vi "DSF.Memory.Pointer.Channel Properties.Read.0D.vi"(8 "error in (no error)":errorcluster, 10 "channel index":u64, 11 "Channel Properties Pointer in":refnum<class "DSF.Memory.Pointer.Channel Properties.lvclass">) -> (0 "error out":errorcluster, 1 "channel properties":T1 {"size" format="%d bytes"; "offset" format="%d bytes"}, 3 "Channel Properties Pointer out":refnum<class "DSF.Memory.Pointer.Channel Properties.lvclass">)   [LabVIEW 2016, in "DSF.Memory.lvlib" / "DSF.Memory.Pointer.Channel Properties.lvclass"]
uses:
  DSF.Memory.Pointer.Channel Properties.lvclass
  C:/Git/SourceTree/DSF/Source/Classes/Memory.Pointer.Array/DSF.Memory.Pointer.Array.lvclass
  C:/Git/SourceTree/DSF/Source/Submodules/Memory Manager/Source/Classes/Pointer/Memory.Pointer.lvclass
  Typedefs/DSF.Common.Channel Properties.ctl
  Typedefs/DSF.Common.DataType.ctl
  Memory.Pointer.Array/DSF.Memory.Pointer.Array.lvclass/DSF.Memory.Pointer.Array.ctl
  Submodules/Memory Manager/Source/Classes/Pointer/Memory.Pointer.lvclass/Memory.Pointer.ctl
  Submodules/Memory Manager/Source/Classes/Pointer/Methods/Memory.Pointer.Errors.vi
  Submodules/Memory Manager/Source/Classes/Pointer/Methods/Memory.Pointer.Errors.Out of Bounds.vi
  Submodules/Memory Manager/Source/Classes/Pointer/Accessors/Get Size.vi
  Submodules/Memory Manager/Source/Submodules/SEH/Source/VIs/Static Error Handling.Source Buffer.Write.String.vi
  Submodules/Memory Manager/Source/Classes/Pointer/Methods/Memory.Pointer.Errors.Write Pointer Size.vi
  Submodules/Memory Manager/Source/Classes/Pointer/Methods/Memory.Pointer.Errors.Create Error.vi
  Submodules/Memory Manager/Source/Submodules/SEH/Source/VIs/Static Error Handling.Source Buffer.Write.Numeric.Scalar.Base10.vi
  Submodules/Memory Manager/Source/Submodules/SEH/Source/VIs/Static Error Handling.Source Buffer.Write.Numeric.Scalar.Base10 (U64).vi
  Submodules/Memory Manager/Source/Submodules/SEH/Source/VIs/Static Error Handling.Error Cluster Constant.vi
  Submodules/Memory Manager/Source/Submodules/SEH/Source/VIs/Static Error Handling.Error Cluster Constant (256B).vi
  Submodules/Memory Manager/Source/Submodules/SEH/Source/VIs/Static Error Handling.Parameters.Status.Set.vi
  Submodules/Memory Manager/Source/Submodules/SEH/Source/VIs/Static Error Handling.Parameters.Code.Set.vi
  Submodules/Memory Manager/Source/Submodules/SEH/Source/VIs/Static Error Handling.Parameters.VI Source.Set.vi
  Submodules/Memory Manager/Source/Constants/Memory.Constants.vi
  Submodules/Memory Manager/Source/Constants/Memory.Constants.Library Name.vi
  Submodules/Memory Manager/Source/Classes/Pointer/Methods/Memory.Pointer.Errors.Get Info.vi
  Memory.Pointer.Array/DSF.Memory.Pointer.Array.lvclass
  Submodules/Memory Manager/Source/Classes/Pointer/Memory.Pointer.lvclass
  DSF.Common.lvlib
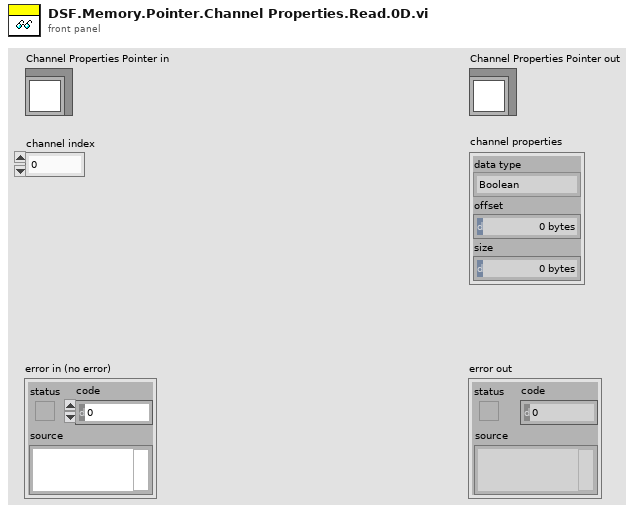
[diagram p1: front panel]
types:
  T1 = typedef "DSF.Common.lvlib/DSF.Common.Channel Properties.ctl" = cluster{"data type":T2, "offset":u64, "size":u64}
  T2 = typedef "DSF.Common.lvlib/DSF.Common.DataType.ctl" = enum8{"Boolean", "Single", "Double", "Int8", "Int16", "Int32", "Int64", "UInt8", "UInt16", "UInt32", "UInt64"}
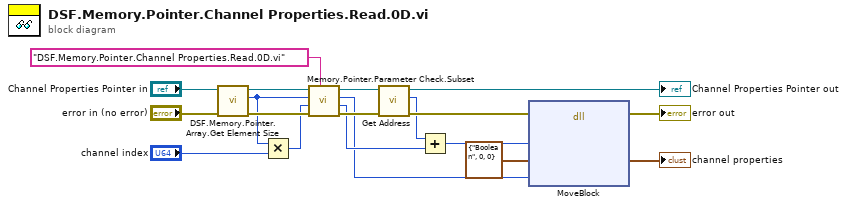
[diagram p0: block diagram]
diagram:
  n1 = call "DSF.Memory.Pointer.Array.Get Element Size.vi"("error in (no error)"="error in (no error)", "Array Pointer in"="Channel Properties Pointer in") -> ("error out"=w8:errorcluster, "element size"=w3:u64, "Array Pointer out"=w9:refnum<class "DSF.Memory.Pointer.Channel Properties.lvclass">)  [unwired: 7 in]
  n2 = Multiply(x=w3, y="channel index") -> (x*y=w4:u64)
  n3 = call "Memory.Pointer.Parameter Check.Subset.vi"("source vi name"="DSF.Memory.Pointer.Channel Properties.Read.0D.vi", "error in (no error)"=w8, "offset (0)"=w4, "length"=w3, "Pointer in"=w9) -> ("error out"=w6:errorcluster, "offset out"=w2:u64, "length"=w1:u64, "Pointer out"=w7:refnum<class "DSF.Memory.Pointer.Channel Properties.lvclass">)  [unwired: 3 in]
  n4 = call "Get Address.vi"("error in (no error)"=w6, "Pointer in"=w7) -> ("error out"=w19:errorcluster, "address"=w15:u64, "Pointer out"=→"Channel Properties Pointer out":refnum<class "DSF.Memory.Pointer.Channel Properties.lvclass">)  [unwired: 7 in]
  n5 = Add(x=w15, y=w2) -> (x+y=w14:u64)
  n6 = dll-call lib="LabVIEW" fn="MoveBlock"(error in=w19, "src"=w14, "dst"=T1 {"data type"=enum."Boolean", "offset"=0, "size"=0} ("Channel Properties"), "size"=w1) -> (error out=→"error out":errorcluster, "dst"=→"channel properties":T1)  [unwired: 5 in, 1 out]
